vi "Command Codes Source.vi"() -> (3 "Commands for FPGA":string[][](table))   [LabVIEW 2013]
panel:
  # "RE-ENTRANT"
  # "SUB-ROUTINE"
  # "Holds the control system commands and info"
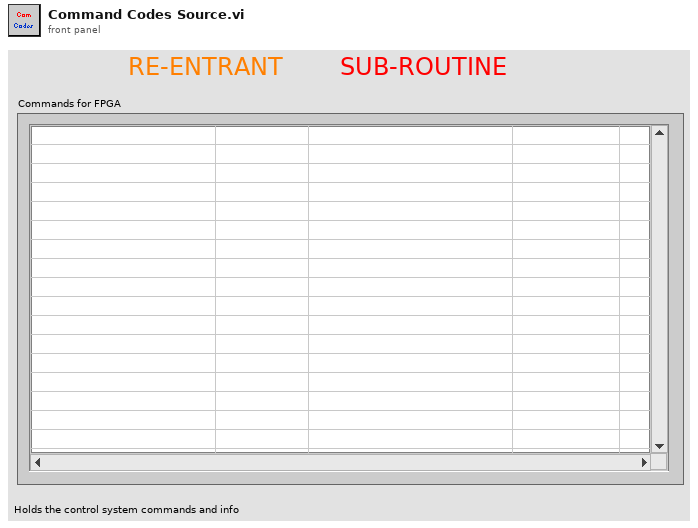
[diagram p1: front panel]
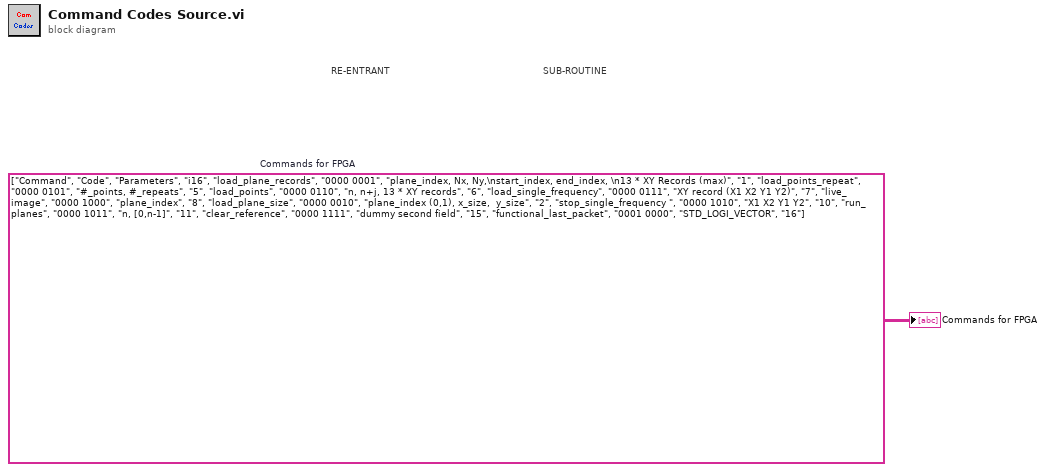
[diagram p0: block diagram]
diagram:
  w1 = string[][] [["Command", "Code", "Parameters", "i16"], ["load_plane_records", "0000 0001", "plane_index, Nx, Ny,\nstart_index, end_index, \n13 * XY Records (max)", "1"], ["load_points_repeat", "0000 0101", "#_points, #_repeats", "5"], ["load_points", "0000 0110", "n, n+j, 13 * XY records", "6"], ["load_single_frequency", "0000 0111", "XY record (X1 X2 Y1 Y2)", "7"], ["live_image", "0000 1000", "plane_index", "8"], ["load_plane_size", "0000 0010", "plane_index (0,1), x_size,  y_size", "2"], ["stop_single_frequency ", "0000 1010", "X1 X2 Y1 Y2", "10"], ["run_planes", "0000 1011", "n, [0,n-1]", "11"], ["clear_reference", "0000 1111", "dummy second field", "15"], ["functional_last_packet", "0001 0000", "STD_LOGI_VECTOR", "16"]]  # Commands for FPGA
  # "SUB-ROUTINE"
  # "RE-ENTRANT"
  "Commands for FPGA" <- w1
